vi "TAT_Com_PLC.vi"() -> ()   [LabVIEW 2017]
uses:
  <vilib>/NI/Modbus Library/API/Wrapper/Create TCP Master.vi
  <vilib>/NI/Modbus Library/API/Master/Modbus Master.lvclass
  <vilib>/NI/Modbus Library/API/Wrapper/API Main.lvlib
panel:
  in  "number of register":u16=4
  in  "starting address":u16=2012
  out "register values":u16[](array[numeric])
  out "Array":i32[](array[numeric])
  out "PLC STATUS":bool
  in  "error in":errorcluster
  in  "stop":bool
  # "Ass & Leak"
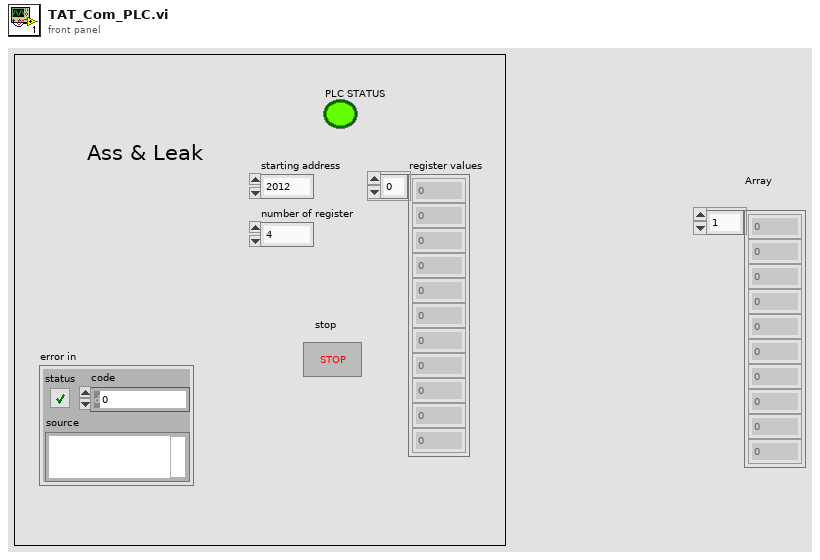
[diagram p1: front panel]
types:
  T1 = enum32{"invalid app kind", "Development System", "Run Time System", "Student Edition", "Embedded LabVIEW", "Evaluation", "Custom"}
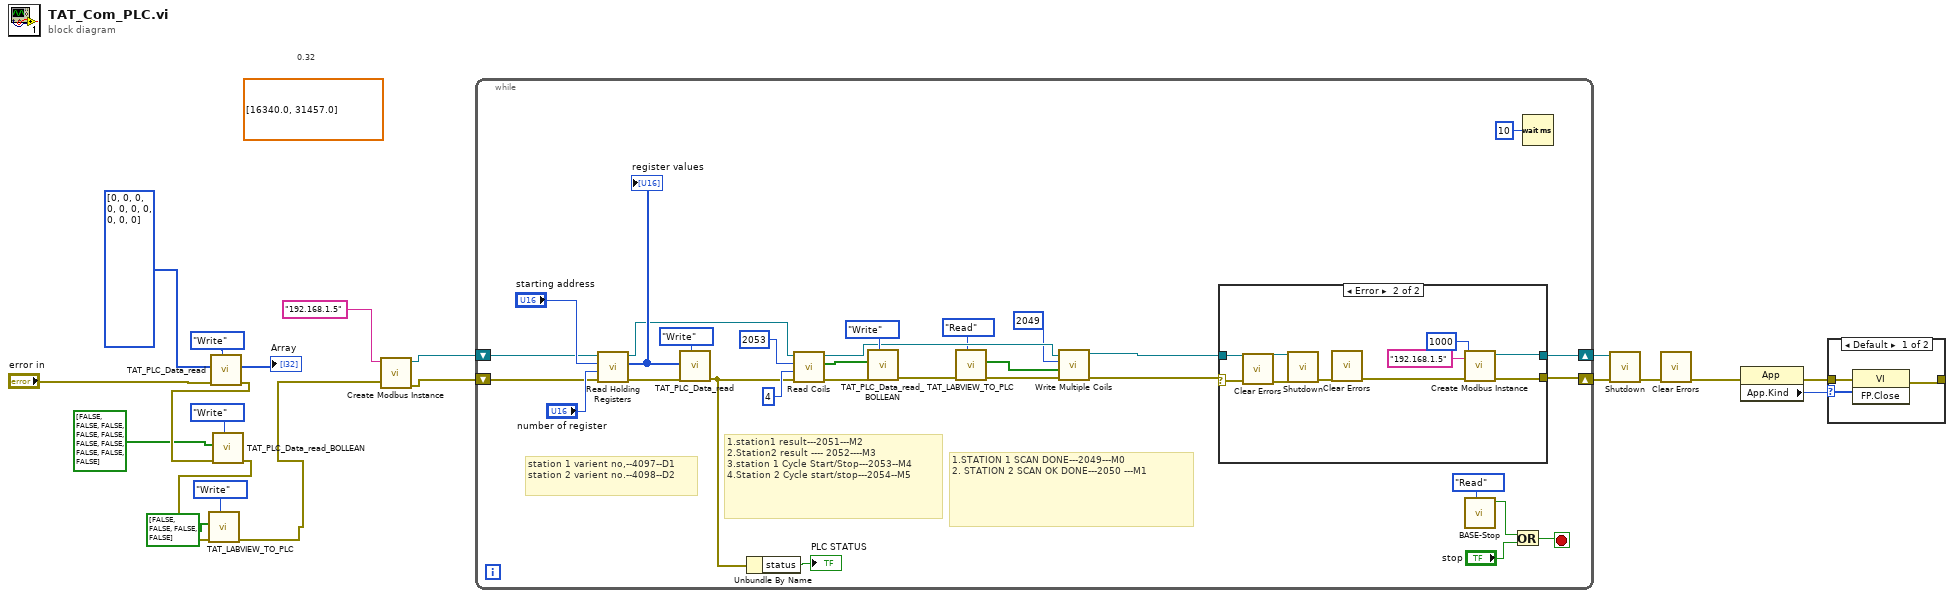
[diagram p0: block diagram]
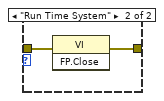
[diagram p3: hidden frame]
diagram:
  (unwired) dbl[] [16340.0, 31457.0] ("register values")
  # "0.32"
  n1 = call "TAT_PLC_Data_read.vi"("Enum"=enum16{"Read", "Write"}."Write", "error in (no error)"="error in", "Array"=i64[] [0, 0, 0, 0, 0, 0, 0, 0, 0, 0] ("Array 3")) -> ("error out"=w8:errorcluster, "Array 2"=→"Array":u16[])  [unwired: 7 in]
  n2 = call "TAT_PLC_Data_read_BOLLEAN.vi"("Enum"=enum16{"Read", "Write"}."Write", "error in (no error)"=w8, "Array"=bool[] [FALSE, FALSE, FALSE, FALSE, FALSE, FALSE, FALSE, FALSE, FALSE, FALSE]) -> ("error out"=w4:errorcluster)  [unwired: 7 in, 1 out]
  n3 = call "TAT_LABVIEW_TO_PLC.vi"("Enum"=enum16{"Read", "Write"}."Write", "error in (no error)"=w4, "Array"=bool[] [FALSE, FALSE, FALSE, FALSE]) -> ("error out"=w5:errorcluster)  [unwired: 7 in, 1 out]
  n4 = call-poly <vilib>:"Create Modbus Instance.vi"("error in"=w5, "address"="192.168.1.5") -> ("error out"=w15:errorcluster, "TCP master instance"=w14:refnum<class "Modbus Master.lvclass">)  [unwired: 8 in]
  n5 = while {
    shift-right: [w48] -> w19
    shift-left: w14 -> [w43]
    shift-right: [w47] -> w18
    shift-left: w15 -> [w44]
    stop <- w49 stop-if-true
    # "1.STATION 1 SCAN DONE---2049---M0\n2. STATION 2 SCAN OK DONE---2050 ---M1"
    # "1.station1 result---2051---M2\n2.Station2 result ---- 2052----M3\n3.station 1 Cycle Start/Stop---2053--M4\n4.Station 2 Cycle start/stop---2054--M5"
    # "station 1 varient no,--4097--D1\nstation 2 varient no.--4098--D2"
    n6 = call-dynamic "Read Holding Registers.vi"("error in"=w44, "number of inputs"="number of register", "starting address"="starting address", "Modbus master in"=w43) -> ("error out"=w38:errorcluster, "register values"=w40:u16[], "Modbus master out"=w34:refnum<class "Modbus Master.lvclass">)  [unwired: 5 in]
    "register values" <- w40
    n7 = call "TAT_PLC_Data_read.vi"("Enum"=enum16{"Read", "Write"}."Write", "error in (no error)"=w38, "Array"=w40) -> ("error out"=w35:errorcluster)  [unwired: 7 in, 1 out]
    n8 = Unbundle By Name(w35) -> ("status"=→"PLC STATUS":bool)
    n9 = call-dynamic "Read Coils.vi"("error in"=w35, "number of inputs"=u16 4, "starting address"=u16 2053, "Modbus master in"=w34) -> ("error out"=w31:errorcluster, "coils"=w33:bool[], "Modbus master out"=w29:refnum<class "Modbus Master.lvclass">)  [unwired: 5 in]
    n10 = call "TAT_PLC_Data_read_BOLLEAN.vi"("Enum"=enum16{"Read", "Write"}."Write", "error in (no error)"=w31, "Array"=w33) -> ("error out"=w25:errorcluster)  [unwired: 7 in, 1 out]
    n11 = call "TAT_LABVIEW_TO_PLC.vi"("Enum"=enum16{"Read", "Write"}."Read", "error in (no error)"=w25) -> ("error out"=w24:errorcluster, "Array 2"=w26:bool[])  [unwired: 8 in]
    n12 = call-dynamic "Write Multiple Coils.vi"("error in"=w24, "coils to write"=w26, "starting address"=u16 2049, "Modbus master in"=w29) -> ("error out"=w30:errorcluster, "Modbus master out"=w28:refnum<class "Modbus Master.lvclass">)  [unwired: 6 in]
    n13 = case shown="Error" w30 {
      selector: w30 -> [w51 w61]
      tunnel: w28 -> [w52 w59]
      tunnel: [w52 w55] -> w48
      tunnel: [w51 w54] -> w47
      frame No Error {
      }
      frame Error {
        n14 = call <vilib>:"Clear Errors.vi"("error in (no error)"=w61) -> ("error out"=w60:errorcluster)  [unwired: 5 in, 1 out]
        n15 = call-dynamic "Shutdown.vi"("error in"=w60, "Modbus master in"=w59) -> ("error out"=w58:errorcluster)  [unwired: 9 in]
        n16 = call <vilib>:"Clear Errors.vi"("error in (no error)"=w58) -> ("error out"=w56:errorcluster)  [unwired: 5 in, 1 out]
        n17 = call-poly <vilib>:"Create Modbus Instance.vi"("error in"=w56, "connect timeout ms"=1000, "address"="192.168.1.5") -> ("error out"=w54:errorcluster, "TCP master instance"=w55:refnum<class "Modbus Master.lvclass">)  [unwired: 7 in]
      }
    }
    n18 = call "BASE-Stop.vi"("Enum"=enum16{"Read", "Write"}."Read") -> ("Stop"=w21:bool)  [unwired: 10 in]
    n19 = Or(x=w21, y="stop") -> (x .or. y?=w49:bool)
    n20 = Wait (ms)(milliseconds to wait=u32 10) -> ()  [unwired: 1 out]
  }
  n21 = call-dynamic "Shutdown.vi"("error in"=w18, "Modbus master in"=w19) -> ("error out"=w2:errorcluster)  [unwired: 9 in]
  n22 = call <vilib>:"Clear Errors.vi"("error in (no error)"=w2) -> ("error out"=w1:errorcluster)  [unwired: 5 in, 1 out]
  n23 = property class="App"(error in=w1) -> (error out=w16:errorcluster, "App.Kind"=w17:T1)  [unwired: 1 in, 1 out]
  n24 = case shown="Default" w17 {
    tunnel: w16 -> [w63 w65]
    tunnel: [w62 w64] -> _
    frame Default {
      n25 = invoke class="VI" method="FP.Close"(error in=w63) -> (error out=w62:errorcluster)  [unwired: 2 in, 2 out]
    }
    frame "Run Time System" {
      n26 = invoke class="VI" method="FP.Close"(error in=w65) -> (error out=w64:errorcluster)  [unwired: 2 in, 2 out]
    }
  }
